vi "Configured Devices UI.vi"(8 "error in (no error)":errorcluster, 11 "HAL Editor in":refnum<class "HAL Editor.lvclass">) -> (0 "error out":errorcluster, 3 "HAL Editor out":refnum<class "HAL Editor.lvclass">)   [LabVIEW 2020, in "HAL Config.lvlib" / "HAL Editor.lvclass"]
uses:
  HAL Editor.lvclass
  HAL Editor.lvclass/HAL Editor.ctl
panel:
  in  "Load INI":bool
  in  "Save INI":bool
  in  "Remove Device":bool
  in  "Edit Device":bool
  in  "New Device":bool
  in  "Device List":i32(listbox)
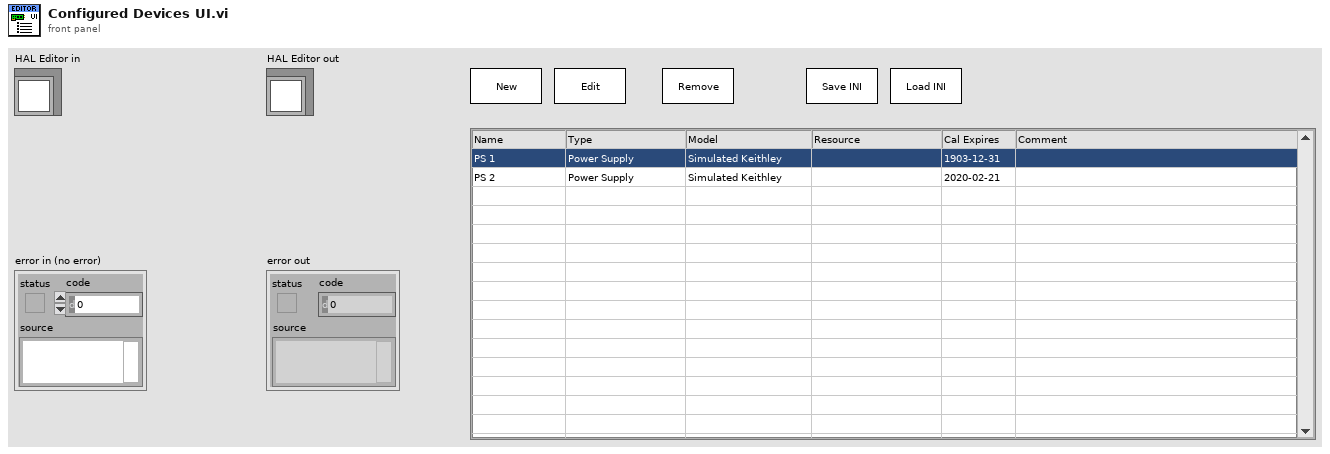
[diagram p1: front panel]
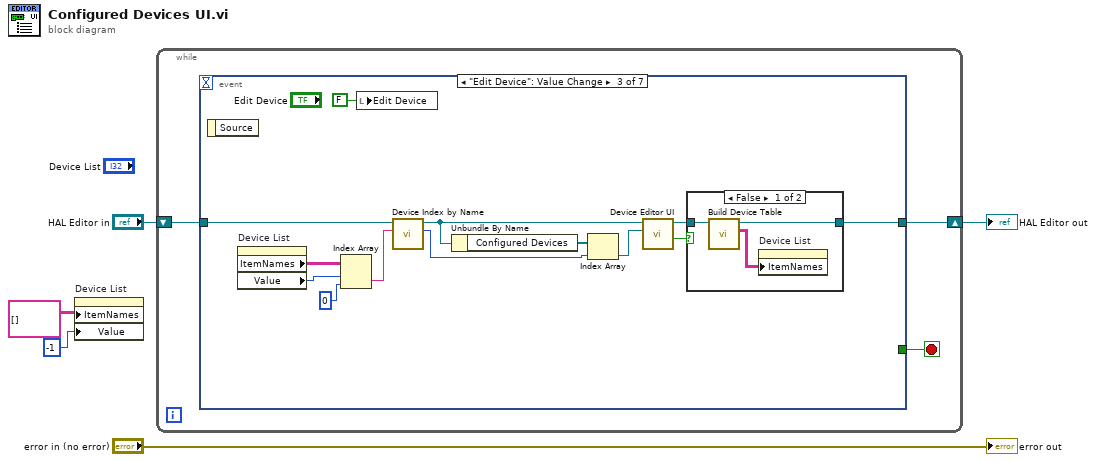
[diagram p0: block diagram]
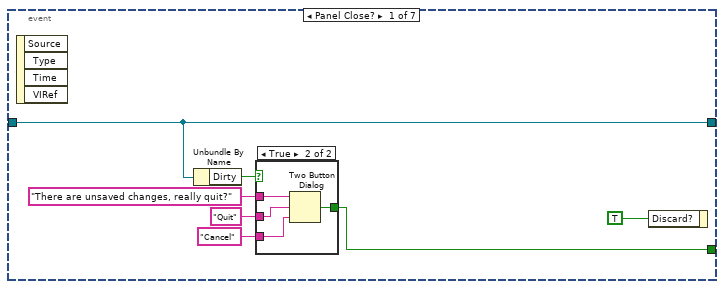
[diagram p2: hidden frame]
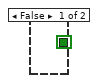
[diagram p3: hidden frame]
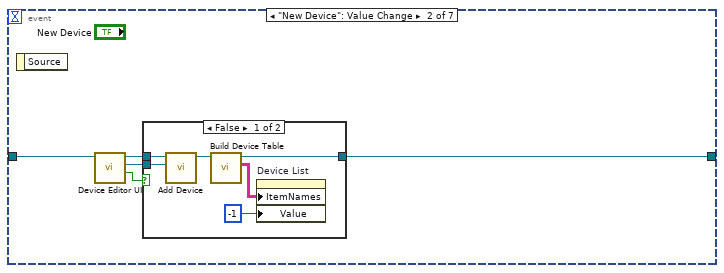
[diagram p4: hidden frame]
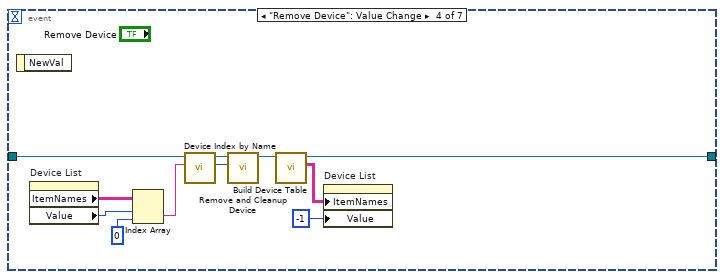
[diagram p7: hidden frame]
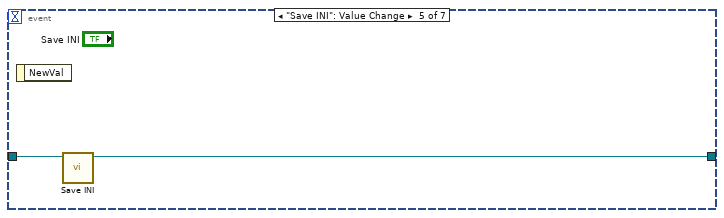
[diagram p8: hidden frame]
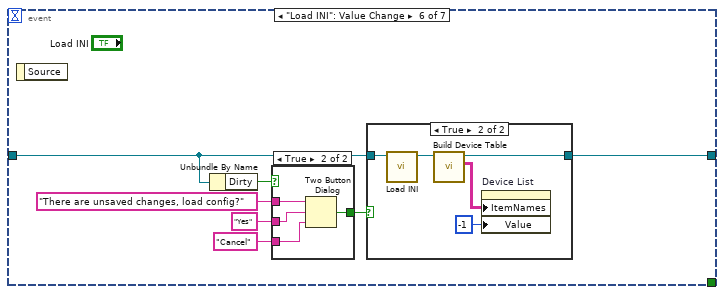
[diagram p9: hidden frame]
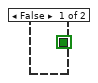
[diagram p11: hidden frame]
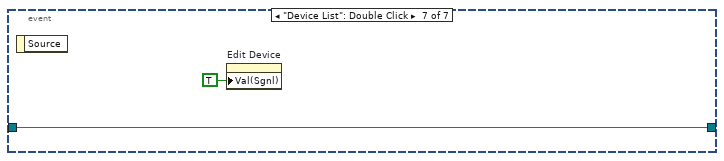
[diagram p12: hidden frame]
diagram:
  n1 = property on="Device List" class="MCListbox (strict)"("ItemNames"=string[][] [] ("Item Names"), "Value"=-1 ("Device List")) -> ()  [unwired: 2 in, 2 out]
  n2 = while {
    shift-right: [w6] -> w3
    shift-left: "HAL Editor in" -> [w7]
    stop <- w8 stop-if-true
    n3 = event shown="[2] \"Edit Device\": Value Change" {
      selector: _ -> [_ _ _ _ _ _ _]
      dyn-events: _ -> [_ _ _ _ _ _ _]
      timeout: _ -> [_ _ _ _ _ _ _]
      tunnel: [w10 _ _ _ _ _ _] -> w8
      tunnel: w7 -> [w14 w25 w36 w50 w62 w64 w82]
      tunnel: [w14 w21 w40 w57 w61 w63 w82] -> w6
      event Panel Close? {
        n4 = event-data() -> ()  [unwired: 1 in, 4 out]
        n5 = Unbundle By Name(w14) -> ("Dirty"=w9:bool)
        n6 = case shown="True" w9 {
          tunnel: "There are unsaved changes, really quit?" -> [_ w20]
          tunnel: "Quit" -> [_ w19]
          tunnel: "Cancel" -> [_ w18]
          tunnel: [TRUE ("T button?") w17] -> w10
          frame False {
          }
          frame True {
            n7 = Two Button Dialog(message=w20, 1:w18, 2:w19) -> (T button?=w17:bool)
          }
        }
        n8 = event-data("Discard?"=TRUE) -> ()  [unwired: 1 in, 1 out]
      }
      event "New Device": Value Change {
        n9 = event-data() -> ()  [unwired: 1 in, 1 out]
        n10 = call "Device Editor UI.vi"("HAL Editor in"=w25) -> ("Cancelled?"=w24:bool, "Updated Device"=w22:refnum<class "Device.lvclass">, "HAL Editor out"=w23:refnum<class "HAL Editor.lvclass">)  [unwired: 7 in, 1 out]
        n11 = case shown="False" w24 {
          tunnel: w23 -> [w31 w32]
          tunnel: w22 -> [w30 _]
          tunnel: [w26 w32] -> w21
          frame False {
            n12 = call "Add Device.vi"("Device"=w30, "HAL Editor in"=w31) -> ("HAL Editor out"=w29:refnum<class "HAL Editor.lvclass">)  [unwired: 8 in, 1 out]
            n13 = call "Build Device Table.vi"("HAL Editor in"=w29) -> ("Device Table"=w27:string[][], "HAL Editor out"=w26:refnum<class "HAL Editor.lvclass">)  [unwired: 8 in, 1 out]
            n14 = property on="Device List" class="MCListbox (strict)"("ItemNames"=w27, "Value"=-1 ("Device List")) -> ()  [unwired: 2 in, 2 out]
          }
          frame True {
          }
        }
      }
      event "Edit Device": Value Change {
        n15 = event-data() -> ()  [unwired: 1 in, 1 out]
        n16 = property on="Device List" class="MCListbox (strict)"() -> ("ItemNames"=w39:string[][], "Value"=w38:i32)  [unwired: 2 in, 2 out]
        n17 = Index Array(array=w39, index (row)=w38, index (col)=0 ("disabled index (col)")) -> (element=w34:string)
        n18 = local write "Edit Device"(FALSE ("Edit Device")) -> ()
        n19 = call "Device Index by Name.vi"("Device Name"=w34, "HAL Editor in"=w36) -> ("Device Index"=w33:i32, "HAL Editor out"=w35:refnum<class "HAL Editor.lvclass">)  [unwired: 7 in, 1 out]
        n20 = Unbundle By Name(w35) -> ("Configured Devices"=w44:refnum<class "Device.lvclass">[])
        n21 = Index Array(array=w44, index=w33) -> (element=w43:refnum<class "Device.lvclass">)
        n22 = call "Device Editor UI.vi"("Device (New)"=w43, "HAL Editor in"=w35) -> ("Cancelled?"=w41:bool, "HAL Editor out"=w42:refnum<class "HAL Editor.lvclass">)  [unwired: 6 in, 2 out]
        n23 = case shown="False" w41 {
          tunnel: w42 -> [w48 w49]
          tunnel: [w46 w49] -> w40
          frame False {
            n24 = call "Build Device Table.vi"("HAL Editor in"=w48) -> ("Device Table"=w47:string[][], "HAL Editor out"=w46:refnum<class "HAL Editor.lvclass">)  [unwired: 8 in, 1 out]
            n25 = property on="Device List" class="MCListbox (strict)"("ItemNames"=w47) -> ()  [unwired: 2 in, 2 out]
          }
          frame True {
          }
        }
      }
      event "Remove Device": Value Change {
        n26 = event-data() -> ()  [unwired: 1 in, 1 out]
        n27 = property on="Device List" class="MCListbox (strict)"() -> ("ItemNames"=w56:string[][], "Value"=w55:i32)  [unwired: 2 in, 2 out]
        n28 = Index Array(array=w56, index (row)=w55, index (col)=0 ("disabled index (col)")) -> (element=w54:string)
        n29 = call "Device Index by Name.vi"("Device Name"=w54, "HAL Editor in"=w50) -> ("Device Index"=w52:i32, "HAL Editor out"=w51:refnum<class "HAL Editor.lvclass">)  [unwired: 7 in, 1 out]
        n30 = call "Remove and Cleanup Device.vi"("Device Index"=w52, "HAL Editor in"=w51) -> ("HAL Editor out"=w60:refnum<class "HAL Editor.lvclass">)  [unwired: 8 in, 1 out]
        n31 = call "Build Device Table.vi"("HAL Editor in"=w60) -> ("Device Table"=w58:string[][], "HAL Editor out"=w57:refnum<class "HAL Editor.lvclass">)  [unwired: 8 in, 1 out]
        n32 = property on="Device List" class="MCListbox (strict)"("ItemNames"=w58, "Value"=-1 ("Device List")) -> ()  [unwired: 2 in, 2 out]
      }
      event "Save INI": Value Change {
        n33 = event-data() -> ()  [unwired: 1 in, 1 out]
        n34 = call "Save INI.vi"("HAL Editor in"=w62) -> ("HAL Editor out"=w61:refnum<class "HAL Editor.lvclass">)  [unwired: 9 in, 1 out]
      }
      event "Load INI": Value Change {
        n35 = event-data() -> ()  [unwired: 1 in, 1 out]
        n36 = Unbundle By Name(w64) -> ("Dirty"=w66:bool)
        n37 = case shown="True" w66 {
          tunnel: "There are unsaved changes, load config?" -> [_ w80]
          tunnel: "Yes" -> [_ w79]
          tunnel: "Cancel" -> [_ w78]
          tunnel: [TRUE ("T button?") w77] -> w65
          frame False {
          }
          frame True {
            n38 = Two Button Dialog(message=w80, 1:w78, 2:w79) -> (T button?=w77:bool)
          }
        }
        n39 = case shown="True" w65 {
          tunnel: w64 -> [w70 w75]
          tunnel: [w70 w73] -> w63
          frame False {
          }
          frame True {
            n40 = call "Load INI.vi"("HAL Editor in"=w75) -> ("HAL Editor out"=w74:refnum<class "HAL Editor.lvclass">)  [unwired: 9 in, 1 out]
            n41 = call "Build Device Table.vi"("HAL Editor in"=w74) -> ("Device Table"=w72:string[][], "HAL Editor out"=w73:refnum<class "HAL Editor.lvclass">)  [unwired: 8 in, 1 out]
            n42 = property on="Device List" class="MCListbox (strict)"("ItemNames"=w72, "Value"=-1 ("Device List")) -> ()  [unwired: 2 in, 2 out]
          }
        }
      }
      event "Device List": Double Click {
        n43 = event-data() -> ()  [unwired: 1 in, 1 out]
        n44 = property on="Edit Device" class="Bool (strict)"("Val(Sgnl)"=TRUE ("Value (Signaling)")) -> ()  [unwired: 2 in, 2 out]
      }
    }
  }
  "HAL Editor out" <- w3
  "error out" <- "error in (no error)"
